vi "Debug VRECT Startup.vi"() -> ()   [LabVIEW 2010]
uses:
  <instrlib>/Keithley 2400/Keithley 24XX.lvlib
panel:
  out "reading":dbl format="%^.2e"
  out "error out":errorcluster
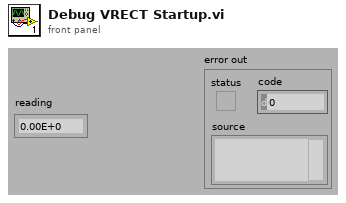
[diagram p1: front panel]
types:
  T1 = enum16{"--Disconnect All--", "Connect PulseGen to CH1", "Connect PulseGen to CH2", "Connect PulseGen to CH3", "Connect PulseGen to CH4", "Connect PulseGen to CH5", "Connect PulseGen to CH6", "Connect PulseGen to CH7", "Connect PulseGen to CH8", "Connect PulseGen to CH9", "Connect PulseGen to CH10", "Connect PulseGen to CH11", "Connect PulseGen to CH12", "Connect PulseGen to CH13", "Connect PulseGen to CH14", "Connect PulseGen to CH15", "Connect PulseGen to CH16", "Connect PulseGen to CH17", "Connect PulseGen to CH18", "Connect PulseGen to CH19", "Connect PulseGen to CH20", "Connect PulseGen to CH21", "Connect PulseGen to CH22", "Connect PulseGen to CH23", "Connect PulseGen to CH24", "Connect PulseGen to CH25", "Set MAG_SW", "Set Dynamic Load", "Set Expansion Trigger", "Trigger Positive Pulse", "Trigger Negative Pulse", "Set MSP Magic Pin", "Set BAT_EN", "Connect MSP_ACLK to CTR", "Connect MSP_MCLK to CTR", "Connect MSP_DIG_TST_OUT to CTR", "Connect STIM_SCK to CTR", "Connect STIM_CLK to CTR", "Connect SMU2 to Magnet", "Magnet Enable", "Cap Short", "Connect Positive Pulse to Pulse Bus", "Connect Negative Pulse to Pulse Bus", "Connect JTAG", "Connect JTAG DVDD Power", "RF Attach", "Connect SMU3 to VBAT", "Connect SMU3 Soft Start", "Connect ARB to Charge Coil", "Connect ARB to Matrix", "Connect CTR to Matrix", "DMM_I Short", "DMM_I 1000 Ohm", "DMM_I 100 Ohm", "DMM_I 10 Ohm", "Connect CH25 to DUT GND"}
  T2 = typedef "niSE SessionRefnum.ctl" = refnum<k1>
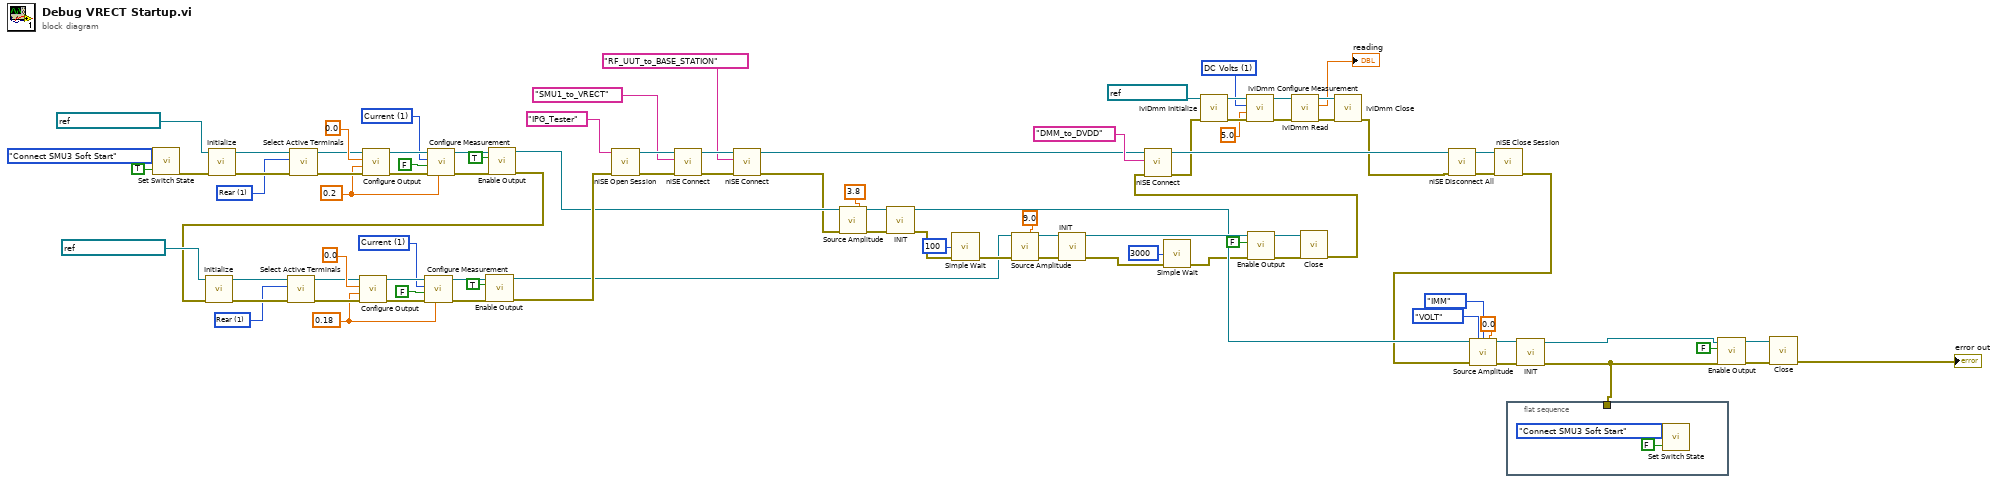
[diagram p0: block diagram]
diagram:
  w42 = u16 1 items=["Volts", "Current", "Resistance"] ("Function (0: Volts)")
  w45 = u16 1 items=["Front", "Rear"] ("Active Terminals (0: Front)")
  w23 = 0.18 ("Compliance  Level (0.1)")
  w55 = u16 1 items=["Volts", "Current", "Resistance"] ("Function (0: Volts)")
  w62 = 1 items=["DC Volts"=1, "AC Volts"=2, "DC Current"=3, "AC Current"=4, "2 Wire Resistance"=5, "4 Wire Resistance"=101, "AC + DC Volts"=106, "AC + DC Current"=107, "Frequency"=104, "Period"=105, "Temperature"=108] ("measurement function (DC Volts)")
  w70 = u16 1 items=["Front", "Rear"] ("Active Terminals (0: Front)")
  w24 = 0.2 ("Compliance  Level (0.1)")
  n1 = call "Set Switch State.vi"("Action"=T1."Connect SMU3 Soft Start", "State"=TRUE) -> ("error out"=w19:errorcluster)  [unwired: 13 in]
  n2 = call <instrlib>:"Initialize.vi"("error in (no error)"=w19, "VISA resource name"=refnum<visa-resource-name> "GPIB0::6::INSTR") -> ("error out"=w72:errorcluster, "VISA resource name out"=w74:refnum<visa-resource-name>)  [unwired: 8 in]
  n3 = call <instrlib>:"Select Active Terminals.vi"("error in (no error)"=w72, "Active Terminals (0: Front)"=w70, "VISA resource name"=w74) -> ("error out"=w71:errorcluster, "VISA resource name out"=w73:refnum<visa-resource-name>)  [unwired: 7 in]
  n4 = call <instrlib>:"Configure Output.vi"("error in (no error)"=w71, "Compliance  Level (0.1)"=w24, "Output Level (0)"=0.0, "VISA resource name"=w73) -> ("error out"=w56:errorcluster, "VISA resource name out"=w57:refnum<visa-resource-name>)  [unwired: 6 in]
  n5 = call <instrlib>:"Configure Measurement.vi"("Manual Range (1.0)"=w24, "error in (no error)"=w56, "Enable Auto Range (T:Enable)"=FALSE, "Function (0: Volts)"=w55, "VISA resource name"=w57) -> ("error out"=w52:errorcluster, "VISA resource name out"=w53:refnum<visa-resource-name>)  [unwired: 5 in]
  n6 = call <instrlib>:"Enable Output.vi"("error in (no error)"=w52, "Enable Output (T: Enable)"=TRUE, "VISA resource name"=w53) -> ("error out"=w22:errorcluster, "VISA resource name out"=w35:refnum<visa-resource-name>)  [unwired: 7 in]
  n7 = call <instrlib>:"Initialize.vi"("error in (no error)"=w22, "VISA resource name"=refnum<visa-resource-name> "GPIB0::9::INSTR") -> ("error out"=w47:errorcluster, "VISA resource name out"=w49:refnum<visa-resource-name>)  [unwired: 8 in]
  n8 = call <instrlib>:"Select Active Terminals.vi"("error in (no error)"=w47, "Active Terminals (0: Front)"=w45, "VISA resource name"=w49) -> ("error out"=w46:errorcluster, "VISA resource name out"=w48:refnum<visa-resource-name>)  [unwired: 7 in]
  n9 = call <instrlib>:"Configure Output.vi"("error in (no error)"=w46, "Compliance  Level (0.1)"=w23, "Output Level (0)"=0.0, "VISA resource name"=w48) -> ("error out"=w43:errorcluster, "VISA resource name out"=w44:refnum<visa-resource-name>)  [unwired: 6 in]
  n10 = call <instrlib>:"Configure Measurement.vi"("Manual Range (1.0)"=w23, "error in (no error)"=w43, "Enable Auto Range (T:Enable)"=FALSE, "Function (0: Volts)"=w42, "VISA resource name"=w44) -> ("error out"=w39:errorcluster, "VISA resource name out"=w40:refnum<visa-resource-name>)  [unwired: 5 in]
  n11 = call <instrlib>:"Enable Output.vi"("error in (no error)"=w39, "Enable Output (T: Enable)"=TRUE, "VISA resource name"=w40) -> ("error out"=w37:errorcluster, "VISA resource name out"=w26:refnum<visa-resource-name>)  [unwired: 7 in]
  n12 = call <vilib>:"niSE Open Session.vi"("error in (no error)"=w37, "Virtual Device Name (SwitchConfiguration1)"="IPG_Tester") -> ("error out"=w89:errorcluster, "NISE Session (out)"=w87:T2)  [unwired: 4 in]
  n13 = call <vilib>:"niSE Connect.vi"("error in (no error)"=w89, "Connection Specification (\"\")"="SMU1_to_VRECT" ("Connection Specification (\"\")"), "NISE Session (in)"=w87) -> ("error out"=w4:errorcluster, "NISE Session (out)"=w5:T2)  [unwired: 7 in]
  n14 = call <vilib>:"niSE Connect.vi"("error in (no error)"=w4, "Connection Specification (\"\")"="RF_UUT_to_BASE_STATION" ("Connection Specification (\"\")"), "NISE Session (in)"=w5) -> ("error out"=w3:errorcluster, "NISE Session (out)"=w2:T2)  [unwired: 7 in]
  n15 = call "Source Amplitude.vi"("VISA resource name"=w35, "Source Level"=3.8, "error in (no error)"=w3) -> ("VISA resource name out"=w36:refnum<visa-resource-name>, "error out"=w34:errorcluster)  [unwired: 11 in]
  n16 = call "INIT.vi"("VISA resource name"=w36, "error in (no error)"=w34) -> ("VISA resource name out"=w15:refnum<visa-resource-name>, "error out"=w32:errorcluster)  [unwired: 12 in]
  n17 = call "Simple Wait.vi"("mS"=u32 100, "error in"=w32) -> ("error out"=w27:errorcluster)  [unwired: 12 in, 1 out]
  n18 = call "Source Amplitude.vi"("VISA resource name"=w26, "Source Level"=9.0, "error in (no error)"=w27) -> ("VISA resource name out"=w30:refnum<visa-resource-name>, "error out"=w29:errorcluster)  [unwired: 11 in]
  n19 = call "INIT.vi"("VISA resource name"=w30, "error in (no error)"=w29) -> ("VISA resource name out"=w25:refnum<visa-resource-name>, "error out"=w9:errorcluster)  [unwired: 12 in]
  n20 = call "Simple Wait.vi"("mS"=u32 3000, "error in"=w9) -> ("error out"=w8:errorcluster)  [unwired: 12 in, 1 out]
  n21 = call <instrlib>:"Enable Output.vi"("error in (no error)"=w8, "Enable Output (T: Enable)"=FALSE, "VISA resource name"=w25) -> ("error out"=w79:errorcluster, "VISA resource name out"=w78:refnum<visa-resource-name>)  [unwired: 7 in]
  n22 = call <instrlib>:"Close.vi"("error in (no error)"=w79, "VISA resource name"=w78) -> ("error out"=w7:errorcluster)  [unwired: 9 in]
  n23 = call <vilib>:"niSE Connect.vi"("error in (no error)"=w7, "Connection Specification (\"\")"="DMM_to_DVDD" ("Connection Specification (\"\")"), "NISE Session (in)"=w2) -> ("error out"=w59:errorcluster, "NISE Session (out)"=w83:T2)  [unwired: 7 in]
  n24 = call <vilib>:"IviDmm Initialize.vi"("error in (no error)"=w59, "logical name (\"SampleDmm\")"=refnum<k15> "IVI-KE2000" ("logical name (\"SampleDmm\")")) -> ("error out"=w67:errorcluster, "instrument handle out"=w68:refnum<k15>)  [unwired: 8 in]
  n25 = call <vilib>:"IviDmm Configure Measurement.vi"("error in (no error)"=w67, "range (-1.0: Auto)"=5.0, "measurement function (DC Volts)"=w62, "instrument handle"=w68) -> ("error out"=w65:errorcluster, "instrument handle out"=w66:refnum<k15>)  [unwired: 6 in]
  n26 = call <vilib>:"IviDmm Read.vi"("error in (no error)"=w65, "instrument handle"=w66) -> ("error out"=w63:errorcluster, "reading"=→"reading":dbl, "instrument handle out"=w64:refnum<k15>)  [unwired: 7 in]
  n27 = call <vilib>:"IviDmm Close.vi"("error in (no error)"=w63, "instrument handle"=w64) -> ("error out"=w58:errorcluster)  [unwired: 9 in]
  n28 = call <vilib>:"niSE Disconnect All.vi"("error in (no error)"=w58, "NISE Session (in)"=w83) -> ("error out"=w88:errorcluster, "NISE Session (out)"=w86:T2)  [unwired: 4 in]
  n29 = call <vilib>:"niSE Close Session.vi"("error in (no error)"=w88, "NISE Session (in)"=w86) -> ("error out"=w6:errorcluster)  [unwired: 5 in]
  n30 = call "Source Amplitude.vi"("VISA resource name"=w15, "Source Function"=enum16{"CURR", "VOLT"}."VOLT", "Mode"=enum16{"IMM", "TRIGGERED"}."IMM", "Source Level"=0.0, "error in (no error)"=w6) -> ("VISA resource name out"=w18:refnum<visa-resource-name>, "error out"=w17:errorcluster)  [unwired: 9 in]
  n31 = flat-sequence {
    tunnel: w13 -> [_]
    frame #0 {
      n32 = call "Set Switch State.vi"("Action"=T1."Connect SMU3 Soft Start", "State"=FALSE) -> ()  [unwired: 13 in, 1 out]
    }
  }
  n33 = call "INIT.vi"("VISA resource name"=w18, "error in (no error)"=w17) -> ("VISA resource name out"=w14:refnum<visa-resource-name>, "error out"=w13:errorcluster)  [unwired: 12 in]
  n34 = call <instrlib>:"Enable Output.vi"("error in (no error)"=w13, "Enable Output (T: Enable)"=FALSE, "VISA resource name"=w14) -> ("error out"=w76:errorcluster, "VISA resource name out"=w77:refnum<visa-resource-name>)  [unwired: 7 in]
  n35 = call <instrlib>:"Close.vi"("error in (no error)"=w76, "VISA resource name"=w77) -> ("error out"=→"error out":errorcluster)  [unwired: 9 in]
